vi "PH_gentec_M-Link.Evt Call Set Trigger Source.vi"(0 "i ref in":refnum<vi>, 2 "Instance":string, 3 "Trigger Source Source":T1 items=["Internal", "External"], 5 "error in (no error)":errorcluster) -> (14 "i ref out":refnum<vi>, 19 "error out":errorcluster)   [LabVIEW 2014, in "PH_gentec_M-Link.lvlib"]
doc: "This VI calls a certain Proc Event by a simple call."
uses:
  PH_gentec_M-Link.lvlib
  non_GPL/instr.lib/gentec-M-LINK/Driver/Type Defs/gentec-M-Link.Trigger Source.ctl
  CSCore/CSSystem/CoreLib/CoreLib.int 2 byte array.vi
  CSCore/BaseProcess/BaseProcess.lvlib
  CSCore/CSSystem/CoreLib/CoreLib.lvlib
  non_GPL/instr.lib/gentec-M-LINK/gentec-M-Link - Driver.lvlib
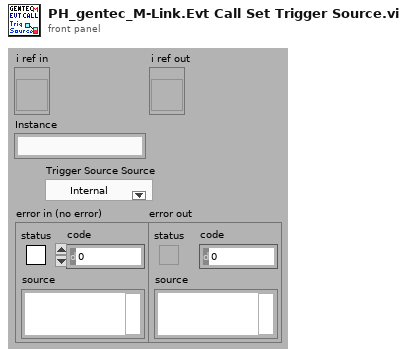
[diagram p1: front panel]
types:
  T1 = typedef "gentec-M-Link - Driver.lvlib/gentec-M-Link.Trigger Source.ctl" = u16
  T2 = typedef "CoreDefs.rawDataType.ctl" = i8[]
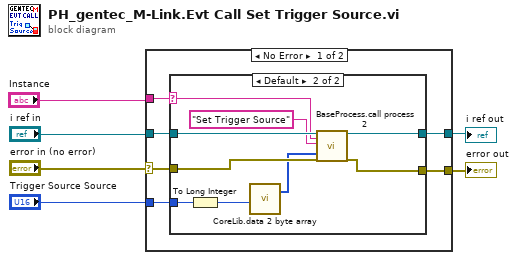
[diagram p0: block diagram]
diagram:
  n1 = case shown="No Error" "error in (no error)" {
    selector: "error in (no error)" -> [w7 w24]
    tunnel: [w12 w25] -> w2
    tunnel: [w11 w24] -> w1
    tunnel: "i ref in" -> [w10 w25]
    tunnel: "Instance" -> [w8 _]
    tunnel: "Trigger Source Source" -> [w9 _]
    frame No Error {
      n2 = case shown="Default" w8 {
        selector: w8 -> [_ w16]
        tunnel: [w14 w23] -> w12
        tunnel: [w13 w22] -> w11
        tunnel: w10 -> [w14 w21]
        tunnel: w7 -> [w13 w20]
        tunnel: w9 -> [_ w18]
        frame "", "N/A" {
        }
        frame Default {
          n3 = To Long Integer(number=w18) -> (32bit integer=w15:i32)
          n4 = call-poly "CoreLib.data 2 byte array.vi"("i32"=w15) -> ("byteArray out"=w17:T2)  [unwired: 18 in]
          n5 = call "BaseProcess.call process 2.vi"("i ref in"=w21, "Object"=w16, "Selector"="Set Trigger Source", "Data"=w17, "error in (no error)"=w20) -> ("i ref out"=w23:refnum<vi>, "error out"=w22:errorcluster)  [unwired: 13 in]
        }
      }
    }
    frame Error {
    }
  }
  "error out" <- w1
  "i ref out" <- w2
